vi "CTRE_CANTalonSRX_SetVoltageRampRate.vi"(8 "error in (no error)":errorcluster, 10 "Throttle Ramp Rate (percent/s)":dbl, 11 "CAN Talon SRX Ref":T1={"DeviceStatus"={"status"=FALSE, "code"=0, "source"=""}, "Type"=enum."PWM", "PWM"={"PWM Channel"=enum."PWM 1", "DeadBand"={"Name"="", "maxPositivePwm"=0, "minPositivePwm"=0, "centerPwm"=0, "maxNegativePwm"=0, "minNegativePwm"=0, "angularRange"=0}}, "CAN"={"Device Number"=0, "SetOutput VI Ref"=variant(enum8{"Percent VBus", "Current", "Speed", "Position", "Voltage"} enum."Percent VBus"), "GetOutput VI Ref"=variant(refnum<k1> refnum), "Enable VI Ref"=variant(dbl 12.0), "Disable VI Ref"=variant(enum8{"Percent VBus", "Speed", "Position", "Slave", "Unchanged / Invalid", "Voltage Compensation", "Current", "Motion Profile"} enum."Percent VBus"), "Data"=variant}, "Invert"=FALSE}) -> (0 "error out":errorcluster, 3 "CAN Talon SRX Ref":T1={"DeviceStatus"={"status"=FALSE, "code"=0, "source"=""}, "Type"=enum."PWM", "PWM"={"PWM Channel"=enum."PWM 1", "DeadBand"={"Name"="", "maxPositivePwm"=0, "minPositivePwm"=0, "centerPwm"=0, "maxNegativePwm"=0, "minNegativePwm"=0, "angularRange"=0}}, "CAN"={"Device Number"=0, "SetOutput VI Ref"=variant(enum8{"Percent VBus", "Current", "Speed", "Position", "Voltage"} enum."Percent VBus"), "GetOutput VI Ref"=variant(refnum<k1> refnum), "Enable VI Ref"=variant(dbl 12.0), "Disable VI Ref"=variant(enum8{"Percent VBus", "Speed", "Position", "Slave", "Unchanged / Invalid", "Voltage Compensation", "Current", "Motion Profile"} enum."Percent VBus"), "Data"=variant}, "Invert"=FALSE})   [LabVIEW 2016]
doc: "Setting the <B>VoltageRampRate (V/s)</B> can be used to limit how quickly the voltage to your motor changes so that you can reduce the current required or make the changes smoother.\n\nIn <B>Percent VBus</B> mode, this is only approximate based on the <B>Max Vout</B> configuration.\n\nThis VI only applies to <B>Percent VBus</B> mode and <B>Voltage</B> mode."
uses:
  <vilib>/Rock Robotics/WPI/MotorControl/WPI_MotorControlDeviceRef.ctl
  <vilib>/Rock Robotics/WPI/MotorControl/WPI_MotorControlType.ctl
  <vilib>/Rock Robotics/SystemInterfaces/DIO/FPGA_DIOPWMChannel.ctl
  <vilib>/Rock Robotics/WPI/PWM/WPI_PWMDeadband.ctl
  <vilib>/Rock Robotics/WPI/ThirdParty/CanMotor/CTRLib-LV-TalonSRX/CTRE_CANTalonSRX_UsageTypes.ctl
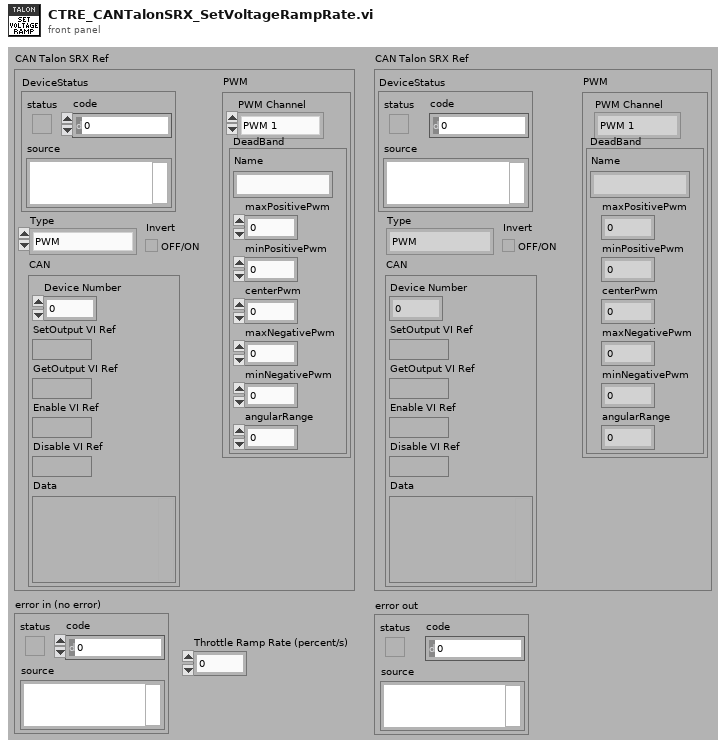
[diagram p1: front panel]
types:
  T1 = typedef "WPI_MotorControlDeviceRef.ctl" = cluster{"DeviceStatus":errorcluster, "Type":T2, "PWM":cluster{"PWM Channel":T3, "DeadBand":T4}, "CAN":cluster{"Device Number":u8, "SetOutput VI Ref":variant, "GetOutput VI Ref":variant, "Enable VI Ref":variant, "Disable VI Ref":variant, "Data":variant}, "Invert":bool}
  T2 = typedef "WPI_MotorControlType.ctl" = enum16{"PWM", "CAN"}
  T3 = typedef "FPGA_DIOPWMChannel.ctl" = enum8{"PWM 0", "PWM 1", "PWM 2", "PWM 3", "PWM 4", "PWM 5", "PWM 6", "PWM 7", "PWM 8", "PWM 9", "PWM MXP 0", "PWM MXP 1", "PWM MXP 2", "PWM MXP 3", "PWM MXP 4", "PWM MXP 5", "PWM MXP 6", "PWM MXP 7", "PWM MXP 8", "PWM MXP 9", "Invalid"}
  T4 = typedef "WPI_PWMDeadband.ctl" = cluster{"Name":string, "maxPositivePwm":i32, "minPositivePwm":i32, "centerPwm":i32, "maxNegativePwm":i32, "minNegativePwm":i32, "angularRange":u16}
  T5 = typedef "CTRE_CANTalonSRX_UsageTypes.ctl" = u32
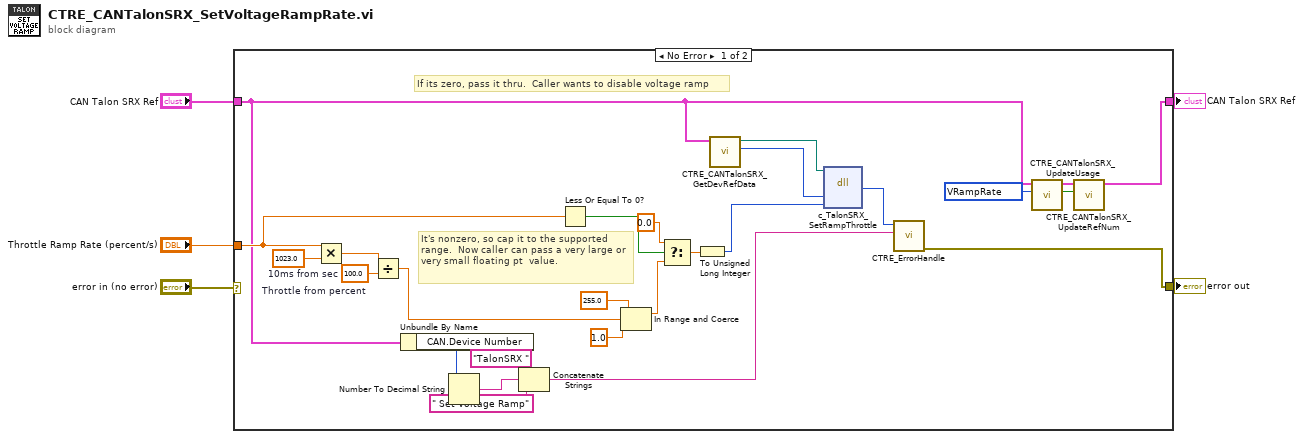
[diagram p0: block diagram]
diagram:
  n1 = case shown="No Error" "error in (no error)" {
    selector: "error in (no error)" -> [_ w33]
    tunnel: [w16 w33] -> w5
    tunnel: [w6 w32] -> w3
    tunnel: "CAN Talon SRX Ref" -> [w10 w32]
    tunnel: "Throttle Ramp Rate (percent/s)" -> [w26 _]
    frame No Error {
      w21 = T5 4194304 items=["Default"=0, "PercentVbus"=1, "Position"=2, "Speed"=4, "Current"=8, "Voltage"=16, "Follower"=32, "MotionProfile"=64, "MotionMagic"=128, "VRampRate"=4194304, "CurrentLimit"=8388608, "ZeroSensorI"=16777216, "ZeroSensorF"=33554432, "ZeroSensorR"=67108864, "ForwardLimitSwitch"=134217728, "ReverseLimitSwitch"=268435456, "ForwardSoftLimit"=536870912, "ReverseSoftLimit"=1073741824, "MultiProfile"=2147483648] ("Usage")
      w29 = 100.0  # 10ms from sec
      w31 = 1023.0  # Throttle from percent
      # "It's nonzero, so cap it to the supported range.  Now caller can pass a very large or very small floating pt  value."
      # "If its zero, pass it thru.  Caller wants to disable voltage ramp"
      n2 = Multiply(x=w26, y=w31) -> (x*y=w30:dbl)
      n3 = Divide(x=w30, y=w29) -> (x/y=w24:dbl)
      n4 = Unbundle By Name(w10) -> ("CAN.Device Number"=w11:u8)
      n5 = Number To Decimal String(number=w11) -> (decimal integer string=w13:string)  [unwired: 1 in]
      n6 = Concatenate Strings("TalonSRX " ("string"), w13, " Set Voltage Ramp" ("string")) -> (w9:string)
      n7 = Less Or Equal To 0?(x=w26) -> (x <= 0?=w28:bool)
      n8 = In Range and Coerce(upper limit=255.0, x=w24, lower limit=1.0) -> (coerced(x)=w23:dbl)  [unwired: 1 out]
      n9 = Select(t=0.0, s=w28, f=w23) -> (s? t:f=w20:dbl)
      n10 = To Unsigned Long Integer(number=w20) -> (unsigned 32bit integer=w17:u32)
      n11 = call <vilib>:"CTRE_CANTalonSRX_GetDevRefData.vi"("MotorControlDevRef"=w10) -> ("handle"=w18:u64, "Library"=w19:path)  [unwired: 6 in, 3 out]
      n12 = dll-call lib="?" fn="c_TalonSRX_SetRampThrottle"(path in=w19, "handle"=w18, "param"=w17) -> ("return type"=w15:i32)  [unwired: 4 in, 2 out]
      n13 = call <vilib>:"CTRE_ErrorHandle.vi"("origin"=w9, "code"=w15) -> ("error out"=w16:errorcluster)  [unwired: 9 in]
      n14 = call <vilib>:"CTRE_CANTalonSRX_UpdateUsage.vi"("Usage"=w21, "CAN Talon SRX Ref"=w10) -> ("Update"=w8:bool, "CAN Talon SRX"=w7:T1)  [unwired: 8 in]
      n15 = call <vilib>:"CTRE_CANTalonSRX_UpdateRefNum.vi"("Update"=w8, "CAN Talon SRX Ref"=w7) -> ("CAN Talon SRX Ref"=w6:T1)  [unwired: 9 in]
    }
    frame Error {
    }
  }
  "CAN Talon SRX Ref" <- w3
  "error out" <- w5
